vi "Test.vi"   [LabVIEW 2021]
uses:
  <vilib>/MediaMongrels Ltd/WebSockets/Sockets/Socket/Socket.lvclass
  <vilib>/MediaMongrels Ltd/WebSockets/WebSockets/WebSocket Server/WebSocket Server.lvclass
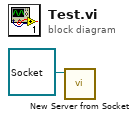
[diagram p0: block diagram]
diagram:
  n1 = call <vilib>:"New Server from Socket.vi"("Socket"=refnum<class "Socket.lvclass"> refnum) -> ()  [unwired: 9 in, 2 out]
